vi "calculaTempoMinimoPraInterceptarBolaEntrandoNaAreaDoGol.vi"(9 "Robot in":T1, 10 "Goleiro.X_padrao":dbl, 11 "IA State":T6={"our_robots"=[], "enemy_robots"=[], "balls"=[], "geometry"={"field_length"=0, "field_width"=0, "goal_width"=0, "goal_depth"=0, "center_circle_radius"=0, "defense_width"=0, "defense_depth"=0, "free_kick_from_defense_dist"=0, "penalty_spot_from_field_line_dist"=0, "penalty_line_from_spot_dist"=0, "half_moon_depth"=0, "half_moon_width"=0}, "IA Judge"={"stage"="", "command"="", "our_goalie_id"=0.0, "enemy_goalie_id"=0.0, "command enum"=enum."Halt", "Time"=enum."Azul"}, "Received Timestamp"=timestamp(0 s since 1904-01-01), "Events"={"Touch"=FALSE, "id touch"=0.0, "Ball out of \nVision"=FALSE, "Ball inside \nGoalie area"=FALSE, "Robot not responding"=FALSE, "Robots responding status"=[1.0, 1.0, 1.0, 1.0, 1.0, 1.0], "Enemy Ball \nPossession"=FALSE, "Id ini Possession"=0.0, "Ball Possesion"=FALSE, "Id Possesion"=0.0, "Ball at\nour goal side"=FALSE, "Ball at\ntouchline"=FALSE, "Ball at\nenemy goal side"=FALSE}}) -> (3 "Tempo_minimo":dbl)   [LabVIEW 2018]
uses:
  Core/AI Input.ctl
  Core/AI Robot.ctl
  Intel/Functions Enum.ctl
  Intel/AttackerStates.ctl
  Path Planning/RRT/PathDests.ctl
  Path Planning/RRT/PathDest.ctl
  Core/AI Ball.ctl
  Core/Field Size.ctl
  Core/AI Judge.ctl
  Intel/Command Enum.ctl
  Util/Events/Events.ctl
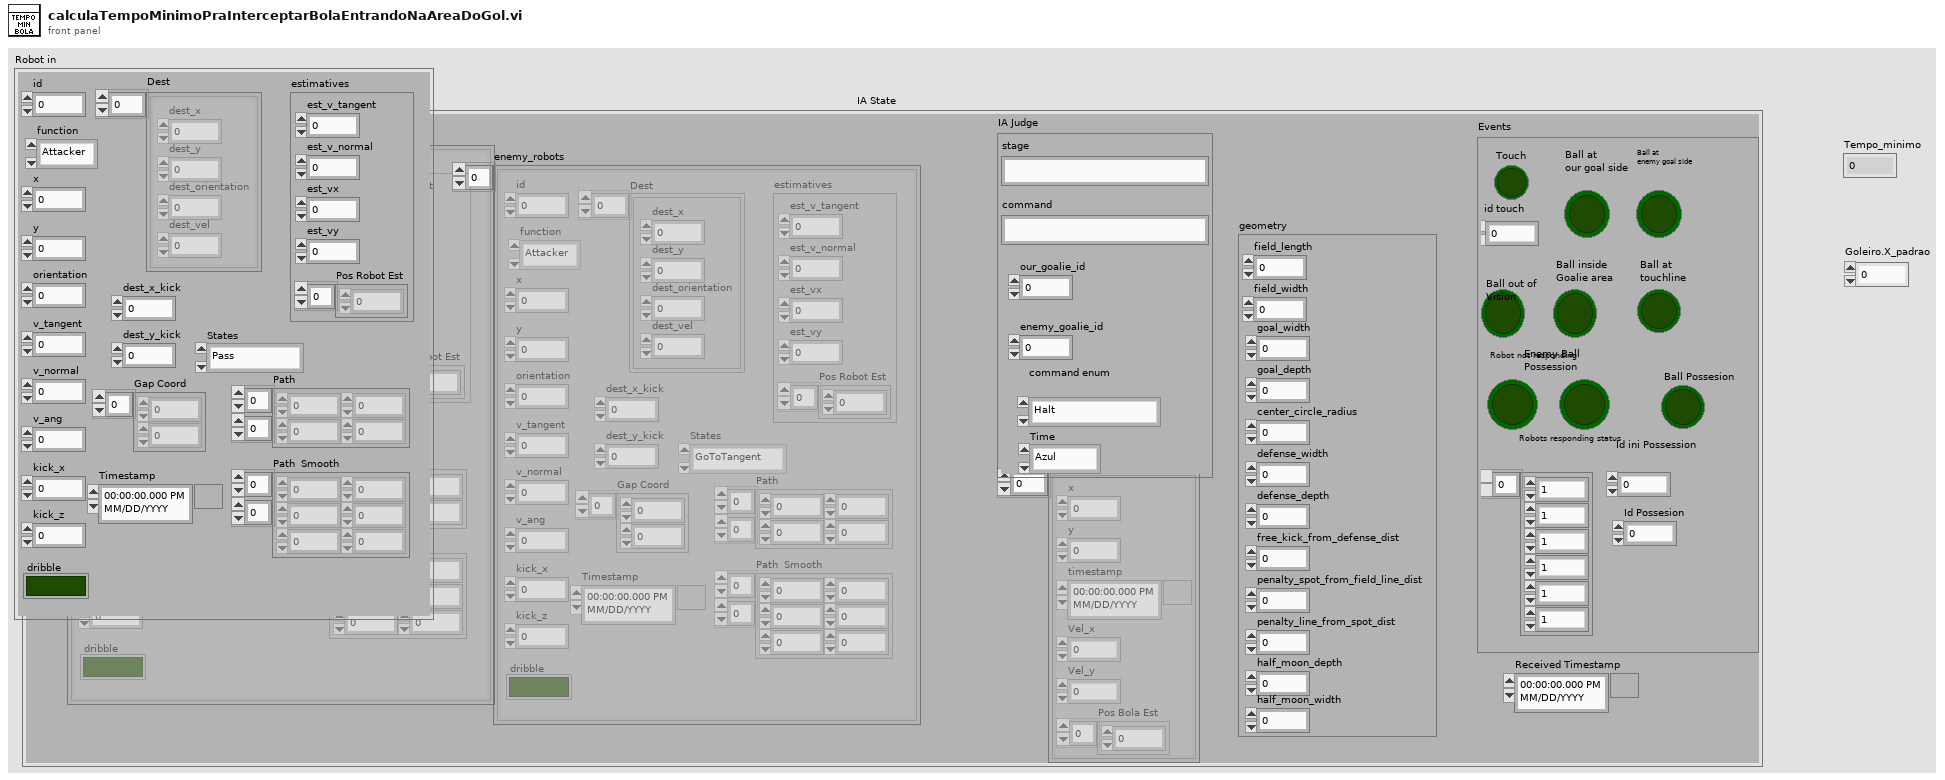
[diagram p1: front panel]
types:
  T1 = typedef "AI Robot.ctl" = cluster{"id":u32, "function":T2, "x":dbl, "y":dbl, "orientation":dbl, "v_tangent":dbl, "v_normal":dbl, "v_ang":dbl, "kick_x":dbl, "kick_z":dbl, "dribble":bool, "Timestamp":timestamp, "estimatives":cluster{"est_v_tangent":dbl, "est_v_normal":dbl, "est_vx":dbl, "est_vy":dbl, "Pos Robot Est":dbl[]}, "dest_x_kick":dbl, "dest_y_kick":dbl, "Gap Coord":dbl[], "States":T3, "Path ":dbl[][], "Path  Smooth":dbl[][], "Dest":T4}
  T2 = typedef "Functions Enum.ctl" = enum16{"Attacker", "Goalie", "Defender", "Striker", "Goto 0", "Dummy", "Kicker", "ZigZag"}
  T3 = typedef "AttackerStates.ctl" = enum16{"Pass", "GoToTangent", "BallGetting", "GoToKick", "Rotate anti-clockwise", "Rotate Clockwise", ""}
  T4 = typedef "PathDests.ctl" = T5[]
  T5 = typedef "PathDest.ctl" = cluster{"dest_x":dbl, "dest_y":dbl, "dest_orientation":dbl, "dest_vel":dbl}
  T6 = typedef "AI Input.ctl" = cluster{"our_robots":T1[], "enemy_robots":T1[], "balls":T7[], "geometry":T8, "IA Judge":T9, "Received Timestamp":timestamp, "Events":T11}
  T7 = typedef "AI Ball.ctl" = cluster{"x":dbl, "y":dbl, "timestamp":timestamp, "Vel_x":dbl, "Vel_y":dbl, "Pos Bola Est":dbl[]}
  T8 = typedef "Field Size.ctl" = cluster{"field_length":u32, "field_width":u32, "goal_width":u32, "goal_depth":u32, "center_circle_radius":u32, "defense_width":u32, "defense_depth":u32, "free_kick_from_defense_dist":u32, "penalty_spot_from_field_line_dist":u32, "penalty_line_from_spot_dist":u32, "half_moon_depth":u32, "half_moon_width":u32}
  T9 = typedef "AI Judge.ctl" = cluster{"stage":string, "command":string, "our_goalie_id":dbl, "enemy_goalie_id":dbl, "command enum":T10, "Time":enum16{"Azul", "Amarelo"}}
  T10 = typedef "Command Enum.ctl" = enum16{"Halt", "Stop", "Force Start", "PKA Normal Start", "Prepare Kickoff Ally", "PKE Normal Start", "Prepare Kickoff Enemy", "Prepare Penalty Ally", "PPA Normal Start", "Prepare Penalty Enemy", "PPE Normal Start", "Ball Placement Enemy Up", "Ball Placement Enemy Down", "Ball Placement Ally Up", "Ball Placement Ally Mid", "Ball Placement Ally Down", "Indirect Free Enemy", "Indirect Free Ally", "Timeout Enemy", "Timeout Ally", "Goal Enemy", "Goal Ally", "Normal Half Time", "Extra Time Break", "Extra Half Time", "None", "Post Game"}
  T11 = typedef "Events.ctl" = cluster{"Touch":bool, "id touch":dbl, "Ball out of \nVision":bool, "Ball inside \nGoalie area":bool, "Robot not responding":bool, "Robots responding status":dbl[], "Enemy Ball \nPossession":bool, "Id ini Possession":dbl, "Ball Possesion":bool, "Id Possesion":dbl, "Ball at\nour goal side":bool, "Ball at\ntouchline":bool, "Ball at\nenemy goal side":bool}
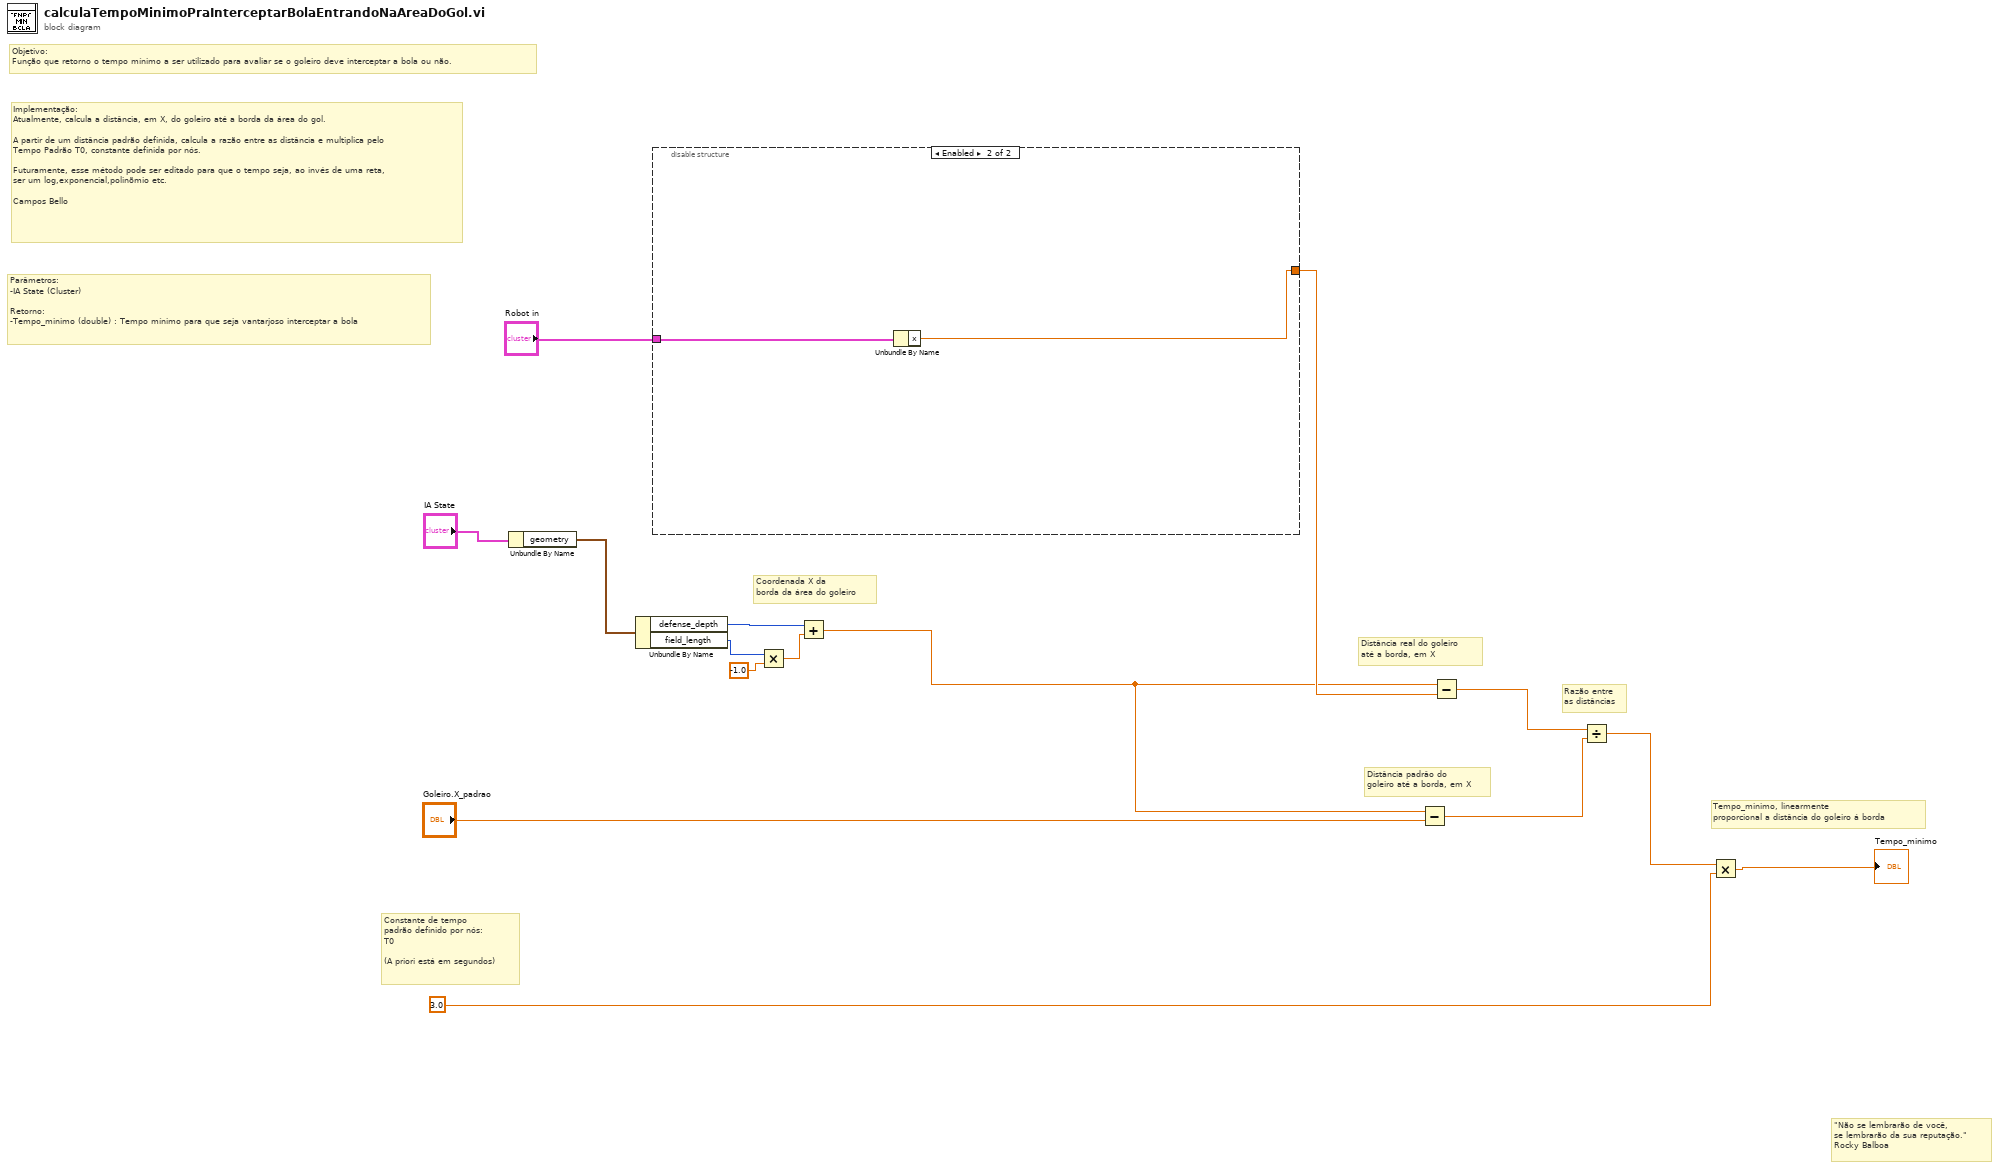
[diagram p0: block diagram]
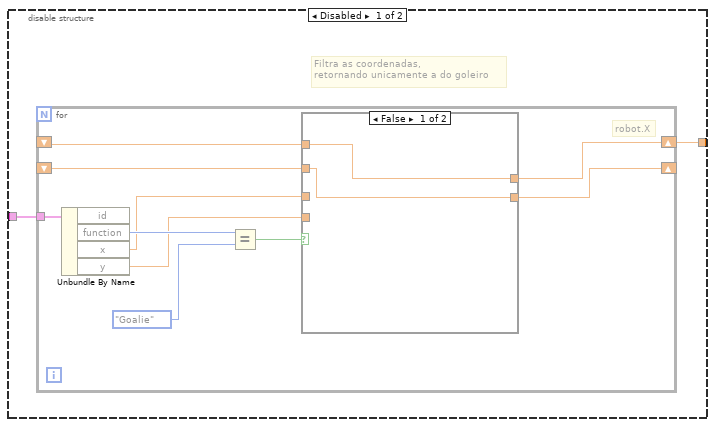
[diagram p2: hidden frame]
diagram:
  # "\"Não se lembrarão de você, \nse lembrarão da sua reputação.\"\nRocky Balboa"
  # "Parâmetros:\n-IA State (Cluster)\n\nRetorno:\n-Tempo_minimo (double) : Tempo mínimo para que seja vantarjoso interceptar a bola"
  # "Implementação: \nAtualmente, calcula a distância, em X, do goleiro até a borda da área do gol.\n\nA partir de um distância padrão definida, calcula a razão entre as distância e multiplica pelo \nTempo Padrão T0, constante definida por nós.\n\nFuturamente, esse método pode ser editado para que o tempo seja, ao invés de uma reta, \nser um log,exponencial,polinõmio etc.\n\nCampos Bello"
  # "Objetivo: \nFunção que retorno o tempo mínimo a ser utilizado para avaliar se o goleiro deve interceptar a bola ou não."
  # "Tempo_minimo, linearmente \nproporcional a distância do goleiro á borda"
  # "Razão entre \nas distâncias"
  # "Distância padrâo do \ngoleiro até a borda, em X"
  # "Constante de tempo \npadrão definido por nós:\nT0\n\n(A priori está em segundos)"
  # "Distância real do goleiro \naté a borda, em X"
  # "Coordenada X da \nborda da área do goleiro"
  n1 = Unbundle By Name("IA State") -> ("geometry"=w14:T8)
  n2 = Unbundle By Name(w14) -> ("defense_depth"=w11:u32, "field_length"=w12:u32)
  n3 = disable-structure shown="Enabled" {
    disable-tunnel: "Robot in" -> [w17 w33]
    disable-tunnel: [w16 w32] -> w9
    frame Disabled {
      # "Filtra as coordenadas, \nretornando unicamente a do goleiro"
      n4 = for {
        tunnel: w17 -> [w27]
        shift-right: [w21] -> w16
        shift-left: _ -> [w19]
        shift-right: [w20] -> _
        shift-left: _ -> [w18]
        # "robot.X"
        n5 = Unbundle By Name(w27) -> ("function"=w26:T2, "x"=w23:dbl, "y"=w22:dbl)  [unwired: 1 out]
        n6 = Equal?(x=w26, y=Functions_Enum."Goalie" ("function")) -> (x = y?=w24:bool)
        n7 = case shown="False" w24 {
          tunnel: w23 -> [_ w31]
          tunnel: w22 -> [_ w30]
          tunnel: [w29 w31] -> w21
          tunnel: [w28 w30] -> w20
          tunnel: w19 -> [w29 _]
          tunnel: w18 -> [w28 _]
          frame False {
          }
          frame True {
          }
        }
      }
    }
    frame Enabled {
      n8 = Unbundle By Name(w33) -> ("x"=w32:dbl)
    }
  }
  n9 = Multiply(x=w12, y=-1.0) -> (x*y=w10:dbl)
  n10 = Add(x=w11, y=w10) -> (x+y=w8:dbl)
  n11 = Subtract(x=w8, y="Goleiro.X_padrao") -> (x-y=w7:dbl)
  n12 = Subtract(x=w8, y=w9) -> (x-y=w6:dbl)
  n13 = Divide(x=w6, y=w7) -> (x/y=w4:dbl)
  n14 = Multiply(x=w4, y=3.0) -> (x*y=→"Tempo_minimo":dbl)
